vi "DegreesToRadians.vi"(1 "Degrees":dbl) -> (0 "Radians":dbl)   [LabVIEW 2009]
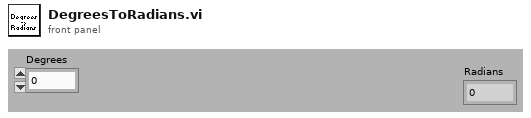
[diagram p1: front panel]
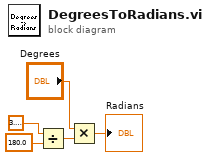
[diagram p0: block diagram]
diagram:
  n1 = Divide(x=3.141592653589793, y=180.0) -> (x/y=w3:dbl)
  n2 = Multiply(x="Degrees", y=w3) -> (x*y=→"Radians":dbl)
